vi "Get Monitor Channel Array.vi"() -> (1 "Channel Array":string[](array[string]))   [LabVIEW 2020, in "afdx_custom_device GUID Utility.lvlib"]
uses:
  afdx_custom_device GUID Utility.lvlib
  Scripting/Constants.vi
  Scripting/afdx_custom_device Scripting.lvlib
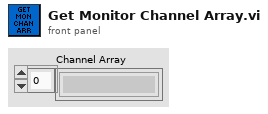
[diagram p1: front panel]
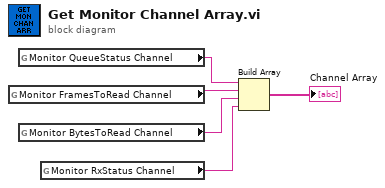
[diagram p0: block diagram]
diagram:
  n1 = global read "Constants.vi" "Monitor FramesToRead Channel"() -> (w5:string)
  n2 = global read "Constants.vi" "Monitor QueueStatus Channel"() -> (w3:string)
  n3 = global read "Constants.vi" "Monitor BytesToRead Channel"() -> (w4:string)
  n4 = global read "Constants.vi" "Monitor RxStatus Channel"() -> (w2:string)
  n5 = Build Array(w3, w5, w4, w2) -> (→"Channel Array":string[])
